vi "FindAllLines.vi"(5 "Reduction loop times":dbl=5.0, 7 "Threshold":dbl=75.0, 8 "Theta Res":dbl=300.0, 9 "raduis thresh":i32=2, 10 "Theta thresh":dbl=0.03, 11 "Image":T1) -> (2 "Lines":cluster{dbl, i32}[](array[cluster]))   [LabVIEW 2012]
uses:
  <vilib>/vision/Image Controls.llb/IMAQ Image.ctl
  <vilib>/vision/NI_Vision_Development_Module.lvlib
panel:
  out "Array":i16[][](array[numeric])
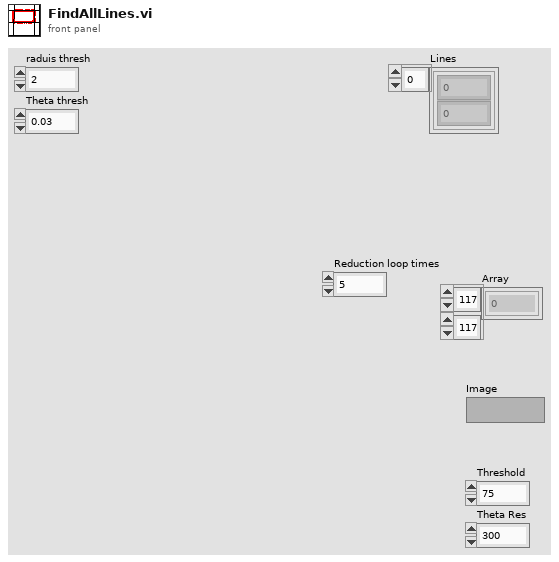
[diagram p1: front panel]
types:
  T1 = typedef "IMAQ Image.ctl" = refnum<image>
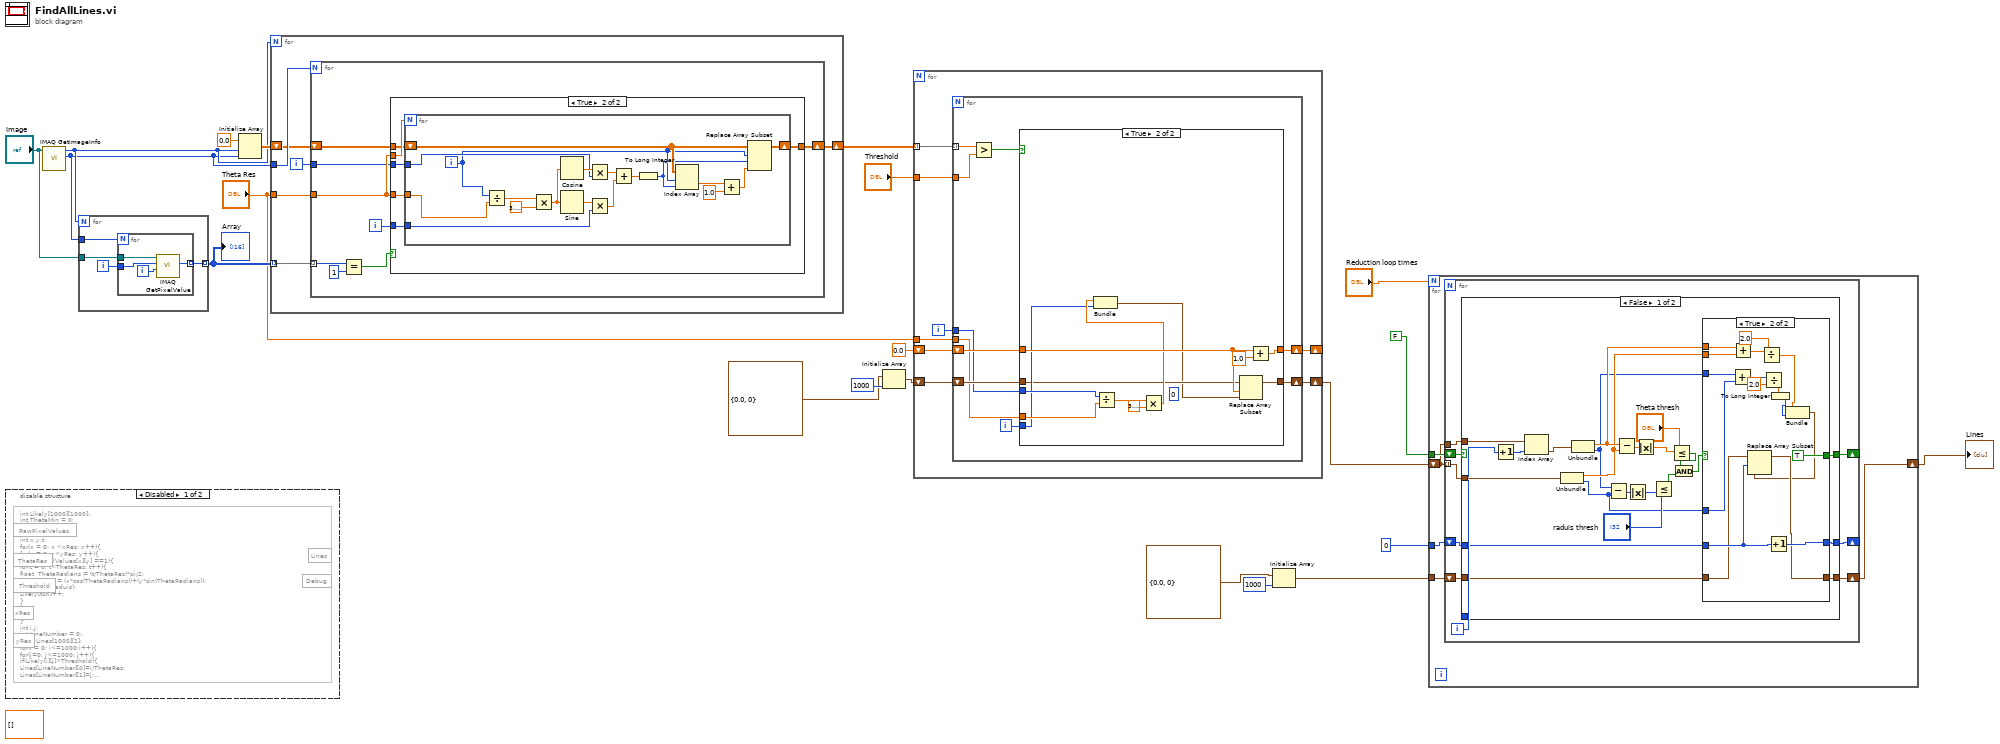
[diagram p0: block diagram]
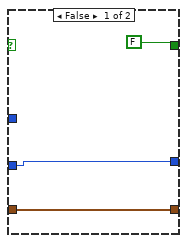
[diagram p2: hidden frame]
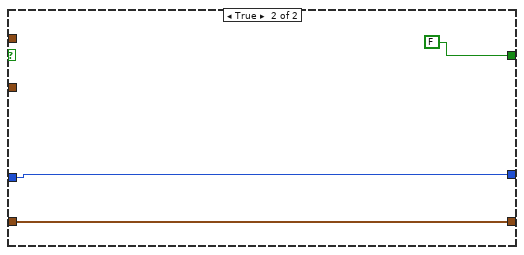
[diagram p3: hidden frame]
diagram:
  (unwired) dbl[][] []
  n1 = disable-structure shown="Disabled" {
    frame Disabled {
      n2 = formula code="int Likely[1000][1000];\nint ThetaMin = 0;\nint Debug;\nDebug =0;\nint x,y,t;\nfor(x = 0; x <xRes; x++){\nfor(y = 0; y<yRes; y++){\nif(RawPixelValues[x][y] ==1){\nfor(t = 0; t<ThetaRes; t++){\nfloat  ThetaRadians = (t/ThetaRes)*pi/2;\nfloat raduis = (x*cos(ThetaRadians))+(y*sin(ThetaRadians));\nint ri = int(raduis);\nLikely[t][ri]++;\n}\n}\n}\n}\nint i,j;\nint LineNumber = 0;\nfloat Lines[1000][1];\nfor(i = 0; i<=1000;i++){\nfor(j=0; j<=1000; j++){\nif(Likely[i][j]>Threshold){\nLines[LineNumber][0]=i/ThetaRes;\nLines[LineNumber][1]=j;\nLineNumber++;\nDebug=j;\n}\n}\n}"() -> ()  [unwired: 5 in, 2 out]
    }
    frame Enabled {
    }
  }
  n3 = call "IMAQ GetImageInfo"("Image"="Image") -> ("Y Resolution"=w10:i32, "X Resolution"=w11:i32)  [unwired: 3 in, 6 out]
  n4 = for {
    N: w11 -> [_]
    tunnel: "Image" -> [w25]
    tunnel: w10 -> [w24]
    tunnel: [w22] -> w21 mode=indexing
    i -> [w23]
    n5 = for {
      N: w24 -> [_]
      tunnel: w25 -> [w29]
      tunnel: w23 -> [w28]
      tunnel: [w26] -> w22 mode=indexing
      i -> [w27]
      n6 = call "IMAQ GetPixelValue"("Image"=w29, "X Coordinate"=w28, "Y Coordinate"=w27) -> ("Pixel Value (I16)"=w26:i16)  [unwired: 3 in, 4 out]
    }
  }
  "Array" <- w21
  n7 = Initialize Array(0.0 ("element"), w11, w10) -> (w17:dbl[][])
  n8 = for {
    N: w11 -> [_]
    tunnel: w10 -> [w35]
    tunnel: w21 -> [w34] mode=indexing
    tunnel: "Theta Res" -> [w33]
    shift-right: [w30] -> w20
    shift-left: w17 -> [w31]
    i -> [w32]
    n9 = for {
      N: w35 -> [_]
      tunnel: w34 -> [w41] mode=indexing
      tunnel: w33 -> [w40]
      tunnel: w32 -> [w39]
      shift-right: [w36] -> w30
      shift-left: w31 -> [w37]
      i -> [w38]
      n10 = Equal?(x=w41, y=i16 1) -> (x = y?=w42:bool)
      n11 = case shown="True" w42 {
        tunnel: w40 -> [_ w50]
        tunnel: w40 -> [_ w49]
        tunnel: w39 -> [_ w48]
        tunnel: w38 -> [_ w47]
        tunnel: w37 -> [w44 w46]
        tunnel: [w44 w45] -> w36
        frame False {
        }
        frame True {
          n12 = for {
            N: w50 -> [_]
            tunnel: w49 -> [w54]
            tunnel: w48 -> [w63]
            tunnel: w47 -> [w62]
            shift-right: [w57] -> w45
            shift-left: w46 -> [w59]
            i -> [w52]
            n13 = Divide(x=w52, y=w54) -> (x/y=w53:dbl)
            n14 = Multiply(x=w53, y=3.141592653589793) -> (x*y=w68:dbl)
            n15 = Cosine(x=w68) -> (cos(x)=w67:dbl)
            n16 = Sine(x=w68) -> (sin(x)=w66:dbl)
            n17 = Multiply(x=w67, y=w63) -> (x*y=w65:dbl)
            n18 = Multiply(x=w66, y=w62) -> (x*y=w64:dbl)
            n19 = Add(x=w65, y=w64) -> (x+y=w56:dbl)
            n20 = To Long Integer(number=w56) -> (32bit integer=w55:i32)
            n21 = Index Array(array=w59, index (row)=w52, index (col)=w55) -> (element=w61:dbl)
            n22 = Add(x=w61, y=1.0) -> (x+y=w58:dbl)
            n23 = Replace Array Subset(array=w59, new element=w58, index (row)=w52, index (col)=w55) -> (w57:dbl[][])
          }
        }
      }
    }
  }
  n24 = Initialize Array(cluster{dbl, i32} {0.0, 0}, 1000 ("dimension size")) -> (w16:cluster{dbl, i32}[])
  n25 = for {
    tunnel: w20 -> [w76] mode=indexing
    tunnel: "Threshold" -> [w75]
    shift-right: [w72] -> _
    shift-left: 0.0 -> [w73]
    tunnel: "Theta Res" -> [w70]
    shift-right: [w69] -> w7
    shift-left: w16 -> [w74]
    i -> [w71]
    n26 = for {
      tunnel: w76 -> [w86] mode=indexing
      tunnel: w75 -> [w85]
      shift-right: [w81] -> w72
      shift-left: w73 -> [w82]
      tunnel: w71 -> [w80]
      tunnel: w70 -> [w79]
      shift-right: [w77] -> w69
      shift-left: w74 -> [w83]
      i -> [w78]
      n27 = Greater?(x=w86, y=w85) -> (0:w84:bool)
      n28 = case shown="True" w84 {
        tunnel: w83 -> [w87 w90]
        tunnel: w82 -> [w88 w98]
        tunnel: [w88 w99] -> w81
        tunnel: w80 -> [_ w94]
        tunnel: w79 -> [_ w95]
        tunnel: w78 -> [_ w91]
        tunnel: [w87 w97] -> w77
        frame False {
        }
        frame True {
          (unwired) 0 ("disabled index (col)")
          n29 = Divide(x=w94, y=w95) -> (x/y=w96:dbl)
          n30 = Multiply(x=w96, y=3.141592653589793) -> (x*y=w92:dbl)
          n31 = Bundle(w92, w91) -> (w89:cluster{dbl, i32})  [unwired: 1 in]
          n32 = Replace Array Subset(array=w90, new element=w89, index=w98) -> (w97:cluster{dbl, i32}[])
          n33 = Add(x=w98, y=1.0) -> (x+y=w99:dbl)
        }
      }
    }
  }
  n34 = Initialize Array(cluster{dbl, i32} {0.0, 0}, 1000 ("dimension size")) -> (w2:cluster{dbl, i32}[])
  n35 = for {
    N: "Reduction loop times" -> [_]
    tunnel: FALSE -> [w105]
    tunnel: 0 -> [w104]
    shift-right: [w101] -> w1
    shift-left: w7 -> [w103]
    tunnel: w2 -> [w102]
    n36 = for {
      tunnel: w103 -> [w111] mode=indexing
      tunnel: w103 -> [w114]
      shift-right: [w108] -> _
      shift-left: w105 -> [w112]
      shift-right: [w110] -> _
      shift-left: w104 -> [w109]
      shift-right: [w106] -> w101
      shift-left: w102 -> [w107]
      i -> [w113]
      n37 = case shown="False" w112 {
        tunnel: w114 -> [w137 _]
        tunnel: w113 -> [w129 _]
        tunnel: w111 -> [w135 _]
        tunnel: w109 -> [w128 w159]
        tunnel: [w127 w159] -> w110
        tunnel: [w121 FALSE] -> w108
        tunnel: w107 -> [w120 w158]
        tunnel: [w119 w158] -> w106
        frame False {
          n38 = Increment(x=w129) -> (x+1=w130:i32)
          n39 = Index Array(array=w137, index=w130) -> (element=w136:cluster{dbl, i32})
          n40 = Unbundle(w135) -> (w117:dbl, w115:i32)
          n41 = Unbundle(w136) -> (w118:dbl, w116:i32)
          n42 = Subtract(x=w116, y=w115) -> (x-y=w132:i32)
          n43 = Subtract(x=w118, y=w117) -> (x-y=w134:dbl)
          n44 = Absolute Value(x=w132) -> (abs(x)=w131:i32)
          n45 = Absolute Value(x=w134) -> (abs(x)=w133:dbl)
          n46 = Less Or Equal?(x=w131, y="raduis thresh") -> (x <= y?=w125:bool)
          n47 = Less Or Equal?(x=w133, y="Theta thresh") -> (x <= y?=w126:bool)
          n48 = And(x=w126, y=w125) -> (x .and. y?=w122:bool)
          n49 = case shown="True" w122 {
            tunnel: w128 -> [w139 w155]
            tunnel: [w139 w157] -> w127
            tunnel: [FALSE TRUE] -> w121
            tunnel: w120 -> [w138 w154]
            tunnel: [w138 w153] -> w119
            tunnel: w118 -> [_ w150]
            tunnel: w117 -> [_ w149]
            tunnel: w116 -> [_ w146]
            tunnel: w115 -> [_ w145]
            frame False {
            }
            frame True {
              n50 = Add(x=w146, y=w145) -> (x+y=w148:i32)
              n51 = Add(x=w150, y=w149) -> (x+y=w151:dbl)
              n52 = Divide(x=w151, y=2.0) -> (x/y=w143:dbl)
              n53 = Divide(x=w148, y=2.0) -> (x/y=w144:dbl)
              n54 = Increment(x=w155) -> (x+1=w157:i32)
              n55 = To Long Integer(number=w144) -> (32bit integer=w142:i32)
              n56 = Bundle(w143, w142) -> (w141:cluster{dbl, i32})  [unwired: 1 in]
              n57 = Replace Array Subset(array=w154, new element=w141, index=w155) -> (w153:cluster{dbl, i32}[])
            }
          }
        }
        frame True {
        }
      }
    }
  }
  "Lines" <- w1
